vi "writebinary.vi"(7 "?":u16(ring) items=["extended precision", "double precision", "single precision", "8 bit byte"], 8 "base path":path, 9 "file index":u64, 10 "data column":string, 11 "data":ext[](array[numeric])) -> ()   [LabVIEW 2015]
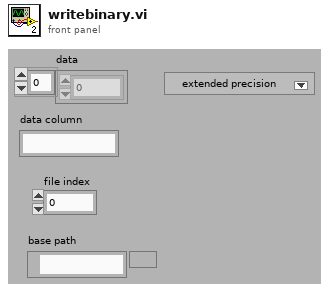
[diagram p1: front panel]
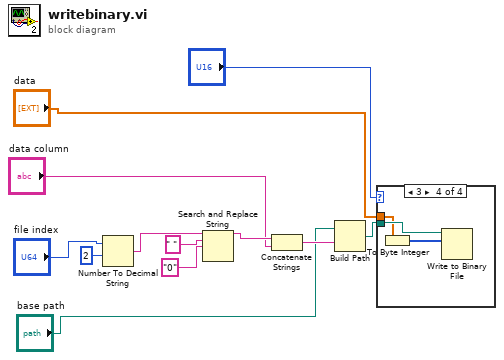
[diagram p0: block diagram]
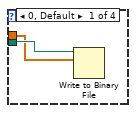
[diagram p2: hidden frame]
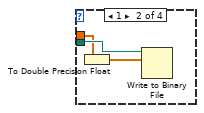
[diagram p3: hidden frame]
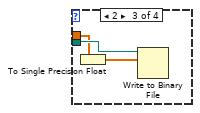
[diagram p4: hidden frame]
diagram:
  n1 = Number To Decimal String(number="file index", width (-)=2) -> (decimal integer string=w8:string)
  n2 = Search and Replace String(input string=w8, search string=" ", replace string="0") -> (result string=w7:string)  [unwired: 2 in, 6 out]
  n3 = Concatenate Strings(w7, "data column") -> (w5:string)
  n4 = Build Path(base path="base path", name or relative path=w5) -> (appended path=w3:path)
  n5 = case shown="3" "?" {
    tunnel: w3 -> [w14 w17 w20 w23]
    tunnel: "data" -> [w13 w16 w19 w22]
    frame 0, Default {
      n6 = Write to Binary File(file (use dialog)=w14, data=w13) -> ()  [unwired: 1 in, 6 out]
    }
    frame 1 {
      n7 = To Double Precision Float(number=w16) -> (double precision float=w15:dbl[])
      n8 = Write to Binary File(file (use dialog)=w17, data=w15) -> ()  [unwired: 1 in, 6 out]
    }
    frame 2 {
      n9 = To Single Precision Float(number=w19) -> (single precision float=w18:sgl[])
      n10 = Write to Binary File(file (use dialog)=w20, data=w18) -> ()  [unwired: 1 in, 6 out]
    }
    frame 3 {
      n11 = To Byte Integer(number=w22) -> (8bit integer=w21:i8[])
      n12 = Write to Binary File(file (use dialog)=w23, data=w21) -> ()  [unwired: 1 in, 6 out]
    }
  }
